vi "set noise2.vi"() -> ()   [LabVIEW 2026]
uses:
  C:/Users/laserfab/Desktop/Cam-PID-LV2026/Thorlabs.MotionControl.Controls.dll
  Thorlabs.MotionControl.Controls.dll
  <vilib>/numeric/Random Number (Range) DBL.vi
  C:/Users/laserfab/Desktop/Cam-PID-LV2026/Thorlabs.MotionControl.TCube.PiezoCLI.dll
  Thorlabs.MotionControl.TCube.PiezoCLI.dll
  <vilib>/ptbypt/NI_PtbyPt.lvlib
panel:
  in  "n millisecondes":u32=100
  out "Tension Y":dbl=50.0
  out "Tension X":dbl=50.0
  in  "Choix Tension Y":T1(ring)=enum."50V"
  in  "Choix Tension X":T1(ring)=enum."50V"
  in  "piezo start":bool
  in  "stop":bool
  out "Graphe Y":cluster{"number":dbl, dbl}(graph)={"number"=50.0, 50.0}
  out "Graphe X":cluster{"number":dbl, dbl}(graph)={"number"=50.0, 50.0}
  in  "Model":T2(ring)
  out "GetOutputVoltage Y":dbl
  out "GetOutputVoltage X":dbl
  in  "TCubePiezoControl 4":refnum<k24>(container)
  in  "SerialNumber Y":string="81844665"
  out "CreateDevice Y":bool
  out "CloseDevice Y":bool
  in  "TCubePiezoControl 3":refnum<k24>(container)
  in  "SerialNumber X":string="81844656"
  out "CreateDevice X":bool
  out "CloseDevice X":bool
  in  "Commande onglets":enum32{"initial", "sin", "gauss"}(tab)
  in  "frequency sin X":dbl=2.0 caption="fréquence" format="%0.2f"
  in  "delta sin X":dbl=1000.0
  out "dt sin X":dbl=7.597
  in  "frequency sin Y":dbl=2.0 caption="fréquence Y" format="%0.2f"
  in  "delta sin Y":dbl=1000.0
  out "dt sin Y":dbl
  in  "dephasage":bool
  in  "-x":dbl=-1.0 format="%#_13g"
  in  "amplitude sin x":dbl=50.0 format="%#_13g"
  in  "amplitude sin y":dbl=50.0 format="%#_13g"
  in  "amplitute target Y":dbl=50.0 format="%#_13g"
  in  "amplitute target X":dbl=50.0 format="%#_13g"
  in  "Offset Gauss X":dbl(knob)=50.0 scale=-50.0..50.0
  in  "Offset Gauss Y":dbl(knob)=50.0 scale=-50.0..50.0
  # "Change Serial Number"
  # "Change Serial Number"
  # "sinus\nX"
  # "sinus\nY"
  # "Gaussien Y"
  # "Gaussien X"
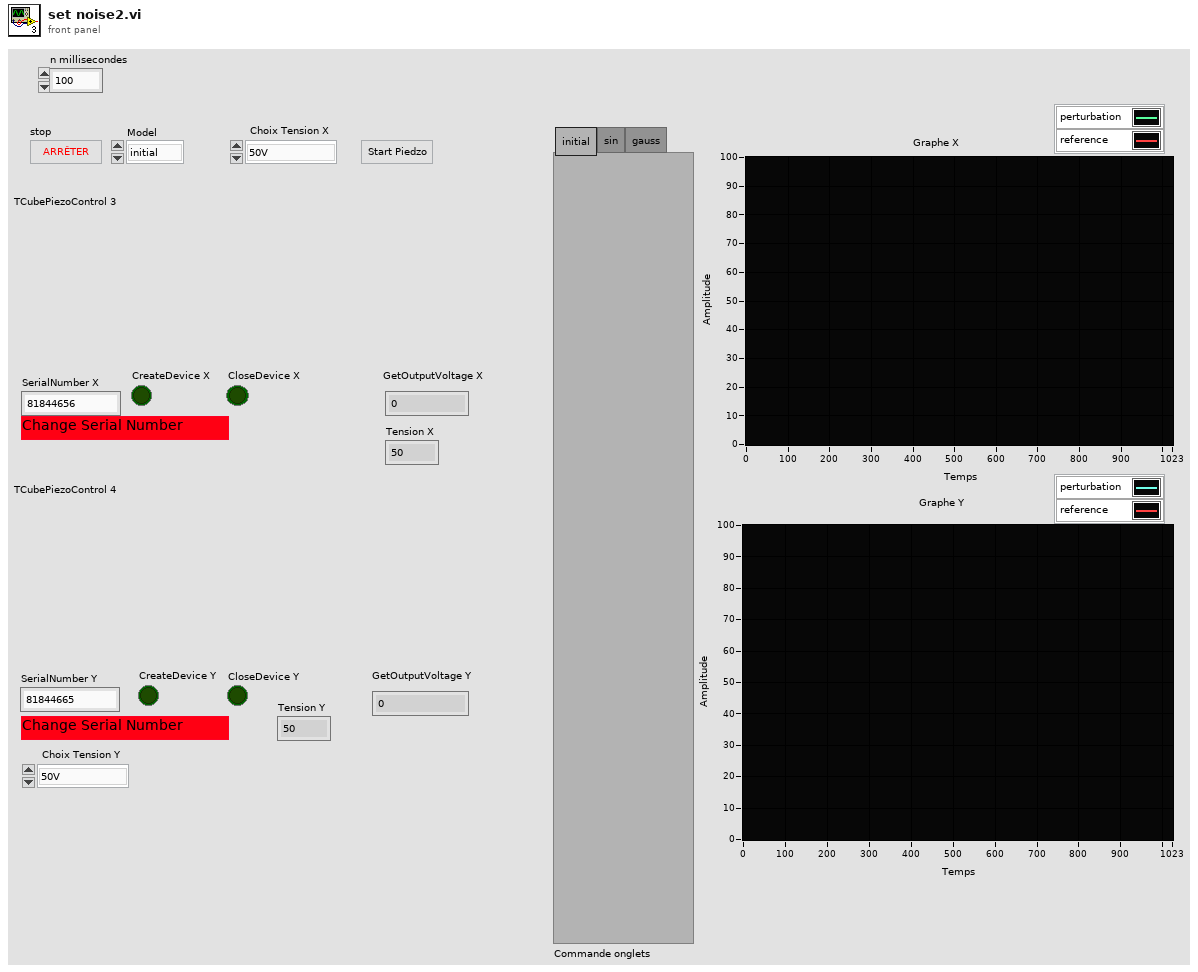
[diagram p1: front panel]
types:
  T1 = enum16{"0V", "10V", "20V", "30V", "40V", "50V", "60V", "70V", "80V", "90V", "100V"}
  T2 = enum16{"initial", "aléatoire", "gaussien", "sinus"}
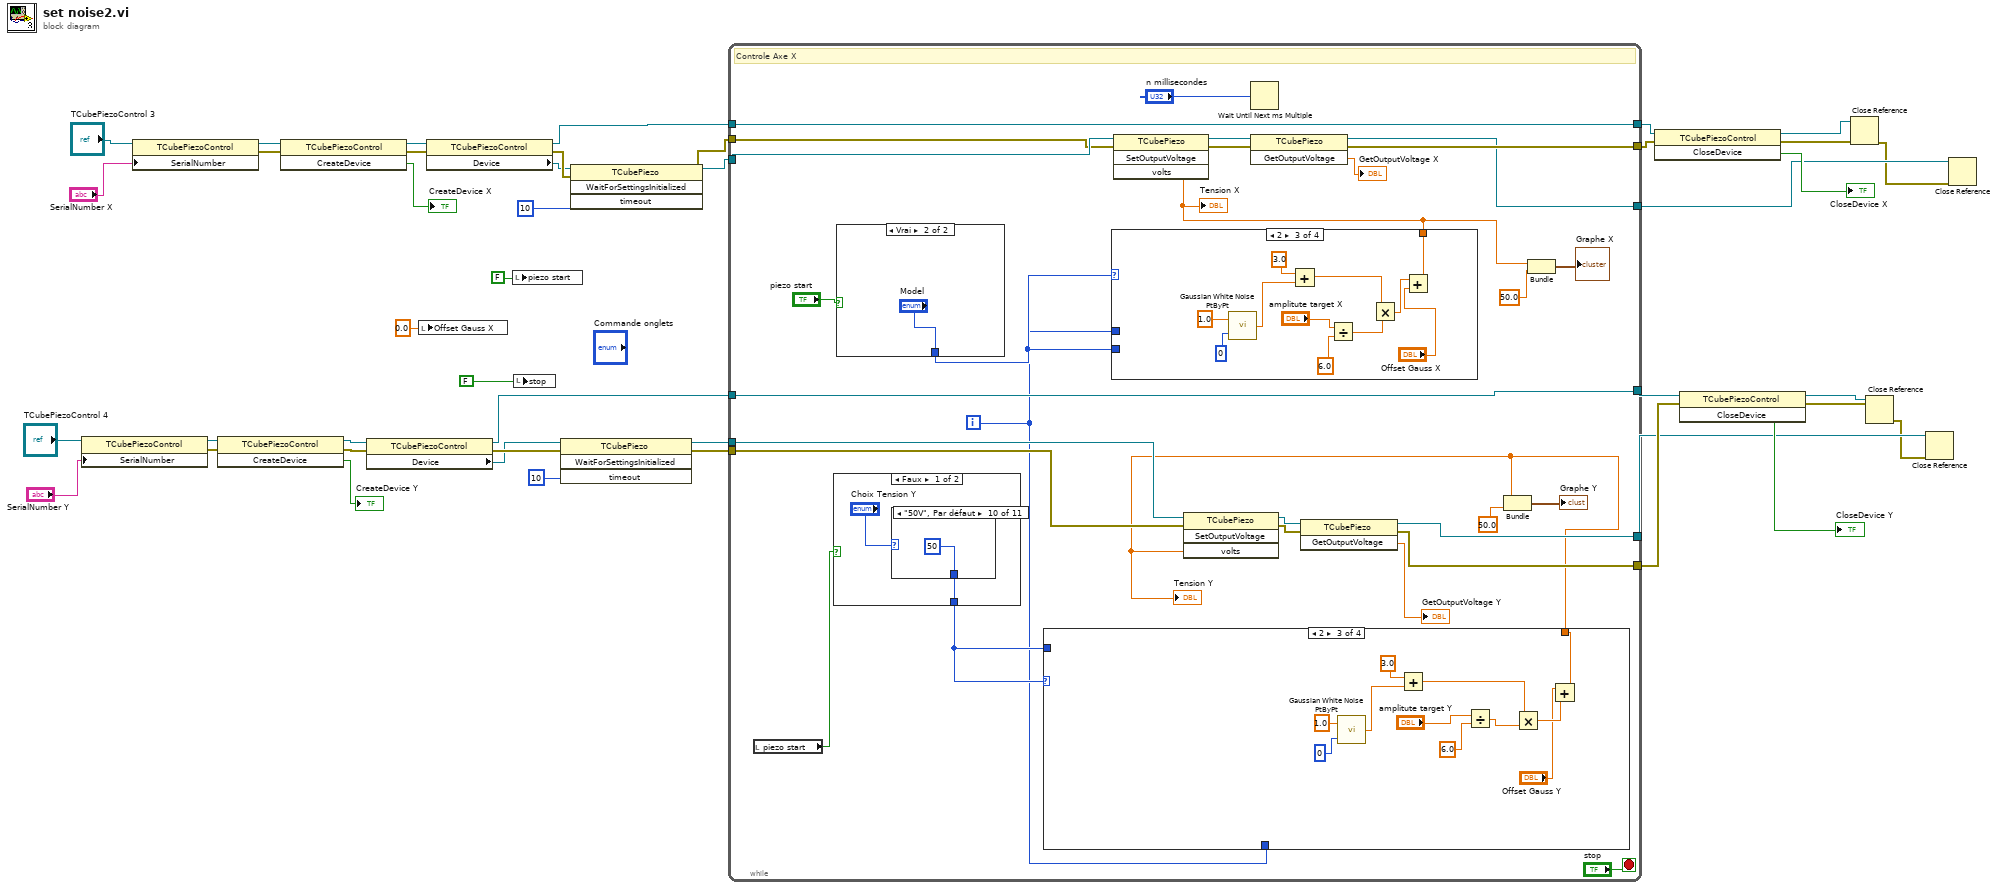
[diagram p0: block diagram]
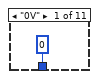
[diagram p2: hidden frame]
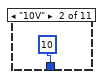
[diagram p3: hidden frame]
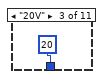
[diagram p4: hidden frame]
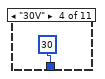
[diagram p5: hidden frame]
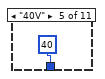
[diagram p6: hidden frame]
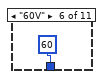
[diagram p7: hidden frame]
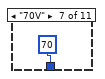
[diagram p8: hidden frame]
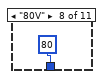
[diagram p9: hidden frame]
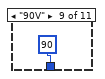
[diagram p10: hidden frame]
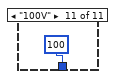
[diagram p11: hidden frame]
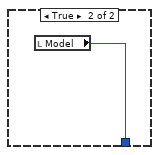
[diagram p12: hidden frame]
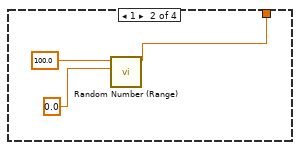
[diagram p14: hidden frame]
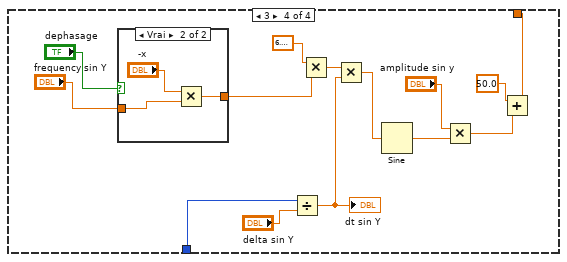
[diagram p15: hidden frame]
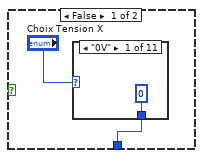
[diagram p17: hidden frame]
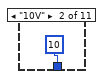
[diagram p18: hidden frame]
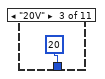
[diagram p19: hidden frame]
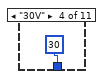
[diagram p20: hidden frame]
diagram:
  n1 = property on="Nœud de propriété" class="TCubePiezoControl"(reference="TCubePiezoControl 4", "SerialNumber"="SerialNumber Y") -> (reference out=w19:refnum<k24>, error out=w20:errorcluster)  [unwired: 1 in]
  n2 = property on="Nœud de propriété" class="TCubePiezoControl"(reference="TCubePiezoControl 3", "SerialNumber"="SerialNumber X") -> (reference out=w32:refnum<k24>, error out=w33:errorcluster)  [unwired: 1 in]
  n3 = invoke on="Nœud de méthode" class="TCubePiezoControl" method="CreateDevice"(reference=w19, error in=w20) -> (reference out=w22:refnum<k24>, error out=w21:errorcluster, "CreateDevice"=→"CreateDevice Y":bool)  [unwired: 1 in]
  n4 = invoke on="Nœud de méthode" class="TCubePiezoControl" method="CreateDevice"(reference=w32, error in=w33) -> (reference out=w35:refnum<k24>, error out=w34:errorcluster, "CreateDevice"=→"CreateDevice X":bool)  [unwired: 1 in]
  n5 = property on="Nœud de propriété" class="TCubePiezoControl"(reference=w22, error in=w21) -> (reference out=w13:refnum<k24>, error out=w25:errorcluster, "Device"=w24:refnum<k24>)
  n6 = local write "Offset Gauss X"(0.0 ("Offset Gauss X")) -> ()
  n7 = property on="Nœud de propriété" class="TCubePiezoControl"(reference=w35, error in=w34) -> (reference out=w37:refnum<k24>, error out=w40:errorcluster, "Device"=w39:refnum<k24>)
  n8 = local write "piezo start"(FALSE ("piezo start")) -> ()
  n9 = local write "stop"(FALSE ("stop")) -> ()
  n10 = invoke on="Nœud de méthode" class="TCubePiezo" method="WaitForSettingsInitialized"(reference=w24, error in=w25, "timeout"=10) -> (reference out=w12:refnum<k24>, error out=w14:errorcluster)  [unwired: 1 in, 2 out]
  n11 = invoke on="Nœud de méthode" class="TCubePiezo" method="WaitForSettingsInitialized"(reference=w39, error in=w40, "timeout"=10) -> (reference out=w42:refnum<k24>, error out=w43:errorcluster)  [unwired: 1 in, 2 out]
  n12 = while {
    tunnel: w37 -> [w72]
    tunnel: [w72] -> w27
    tunnel: [w71] -> w38
    tunnel: w42 -> [w68]
    tunnel: w43 -> [w67]
    tunnel: w14 -> [w51]
    tunnel: [w50] -> w6
    tunnel: w13 -> [w50]
    tunnel: w12 -> [w49]
    tunnel: [w48] -> w5
    tunnel: [w47] -> w9
    tunnel: [w46] -> w4
    i -> [w44]
    stop <- "stop" stop-if-true
    # "Controle Axe X"
    n13 = local read "piezo start"() -> (w58:bool)
    n14 = case shown="Faux" w58 {
      tunnel: [w74 w86] -> w57
      frame False {
        n15 = case shown="\"50V\", Par défaut" "Choix Tension Y" {
          tunnel: [0 10 20 30 40 60 70 80 90 50 100] -> w74
          frame "0V" {
          }
          frame "10V" {
          }
          frame "20V" {
          }
          frame "30V" {
          }
          frame "40V" {
          }
          frame "60V" {
          }
          frame "70V" {
          }
          frame "80V" {
          }
          frame "90V" {
          }
          frame "50V", Default {
          }
          frame "100V" {
          }
        }
      }
      frame True {
        n16 = local read "Model"() -> (w86:T2)
      }
    }
    n17 = case shown="Vrai" "piezo start" {
      tunnel: [w121 "Model"] -> w63
      frame False {
        n18 = case shown="\"0V\"" "Choix Tension X" {
          tunnel: [0 10 20 30 40 60 70 80 90 50 100] -> w121
          frame "0V" {
          }
          frame "10V" {
          }
          frame "20V" {
          }
          frame "30V" {
          }
          frame "40V" {
          }
          frame "60V" {
          }
          frame "70V" {
          }
          frame "80V" {
          }
          frame "90V" {
          }
          frame "50V", Default {
          }
          frame "100V" {
          }
        }
      }
      frame True {
      }
    }
    n19 = case shown="2" w57 {
      tunnel: [w87 w90 w92 w103] -> w45
      tunnel: w44 -> [_ _ _ w108]
      tunnel: w57 -> [w87 _ _ _]
      frame 0, Default {
      }
      frame 1 {
        n20 = call-poly <vilib>:"Random Number (Range).vi"("lower bound (0)"=0.0, "upper bound (100)"=100.0) -> ("number"=w90:dbl)  [unwired: 9 in]
      }
      frame 2 {
        n21 = call <vilib>:"Gaussian White Noise PtByPt.vi"("seed"=0, "standard deviation"=1.0) -> ("Gaussian white noise"=w99:dbl)  [unwired: 1 in]
        n22 = Add(x=3.0, y=w99) -> (x+y=w98:dbl)
        n23 = Divide(x="amplitute target Y", y=6.0) -> (x/y=w96:dbl)
        n24 = Multiply(x=w98, y=w96) -> (x*y=w93:dbl)
        n25 = Add(x="Offset Gauss Y", y=w93) -> (x+y=w92:dbl)
      }
      frame 3 {
        n26 = case shown="Vrai" "dephasage" {
          tunnel: "frequency sin Y" -> [w116 w119]
          tunnel: [w116 w117] -> w105
          frame False {
          }
          frame True {
            n27 = Multiply(x="-x", y=w119) -> (x*y=w117:dbl)
          }
        }
        n28 = Divide(x=w108, y="delta sin Y") -> (x/y=w112:dbl)
        "dt sin Y" <- w112
        n29 = Multiply(x=6.283185307179586, y=w105) -> (x*y=w110:dbl)
        n30 = Multiply(x=w110, y=w112) -> (x*y=w113:dbl)
        n31 = Sine(x=w113) -> (sin(x)=w104:dbl)
        n32 = Multiply(x="amplitude sin y", y=w104) -> (x*y=w109:dbl)
        n33 = Add(x=50.0, y=w109) -> (x+y=w103:dbl)
      }
    }
    "Tension Y" <- w45
    n34 = case shown="2" w63 {
      tunnel: [w134 w136 w139 w150] -> w61
      tunnel: w44 -> [_ _ _ w153]
      tunnel: w63 -> [w134 _ _ _]
      frame 0, Default {
      }
      frame 1 {
        n35 = call-poly <vilib>:"Random Number (Range).vi"("lower bound (0)"=0.0, "upper bound (100)"=100.0) -> ("number"=w136:dbl)  [unwired: 9 in]
      }
      frame 2 {
        n36 = call <vilib>:"Gaussian White Noise PtByPt.vi"("seed"=0, "standard deviation"=1.0) -> ("Gaussian white noise"=w146:dbl)  [unwired: 1 in]
        n37 = Add(x=3.0, y=w146) -> (x+y=w145:dbl)
        n38 = Divide(x="amplitute target X", y=6.0) -> (x/y=w143:dbl)
        n39 = Multiply(x=w145, y=w143) -> (x*y=w140:dbl)
        n40 = Add(x=w140, y="Offset Gauss X") -> (x+y=w139:dbl)
      }
      frame 3 {
        n41 = Divide(x=w153, y="delta sin X") -> (x/y=w157:dbl)
        "dt sin X" <- w157
        n42 = Multiply(x=6.283185307179586, y="frequency sin X") -> (x*y=w159:dbl)
        n43 = Multiply(x=w159, y=w157) -> (x*y=w156:dbl)
        n44 = Sine(x=w156) -> (sin(x)=w151:dbl)
        n45 = Multiply(x="amplitude sin x", y=w151) -> (x*y=w152:dbl)
        n46 = Add(x=50.0, y=w152) -> (x+y=w150:dbl)
      }
    }
    "Tension X" <- w61
    n47 = invoke on="Nœud de méthode" class="TCubePiezo" method="SetOutputVoltage"(reference=w68, error in=w67, "volts"=w61) -> (reference out=w66:refnum<k24>, error out=w65:errorcluster)  [unwired: 1 in, 2 out]
    n48 = invoke on="Nœud de méthode" class="TCubePiezo" method="SetOutputVoltage"(reference=w49, error in=w51, "volts"=w45) -> (reference out=w54:refnum<k24>, error out=w55:errorcluster)  [unwired: 1 in, 2 out]
    n49 = Wait Until Next ms Multiple(millisecond multiple="n millisecondes") -> ()  [unwired: 1 out]
    n50 = invoke on="Nœud de méthode" class="TCubePiezo" method="GetOutputVoltage"(reference=w66, error in=w65) -> (reference out=w46:refnum<k24>, error out=w71:errorcluster, "GetOutputVoltage"=→"GetOutputVoltage X":dbl)  [unwired: 1 in]
    n51 = invoke on="Nœud de méthode" class="TCubePiezo" method="GetOutputVoltage"(reference=w54, error in=w55) -> (reference out=w48:refnum<k24>, error out=w47:errorcluster, "GetOutputVoltage"=→"GetOutputVoltage Y":dbl)  [unwired: 1 in]
    n52 = Bundle("number"=w45, 50.0) -> (→"Graphe Y":cluster{"number":dbl, dbl})  [unwired: 1 in]
    n53 = Bundle("number"=w61, 50.0) -> (→"Graphe X":cluster{"number":dbl, dbl})  [unwired: 1 in]
  }
  n54 = invoke on="Nœud de méthode" class="TCubePiezoControl" method="CloseDevice"(reference=w27, error in=w38) -> (reference out=w10:refnum<k24>, error out=w7:errorcluster, "CloseDevice"=→"CloseDevice X":bool)  [unwired: 1 in]
  n55 = invoke on="Nœud de méthode" class="TCubePiezoControl" method="CloseDevice"(reference=w6, error in=w9) -> (reference out=w11:refnum<k24>, error out=w8:errorcluster, "CloseDevice"=→"CloseDevice Y":bool)  [unwired: 1 in]
  n56 = Close Reference(reference=w10, error in (no error)=w7) -> (error out=w3:errorcluster)
  n57 = Close Reference(reference=w11, error in (no error)=w8) -> (error out=w2:errorcluster)
  n58 = Close Reference(reference=w5, error in (no error)=w2) -> ()  [unwired: 1 out]
  n59 = Close Reference(reference=w4, error in (no error)=w3) -> ()  [unwired: 1 out]
